vi "Realtime Curve Fitting.vi"() -> ()   [LabVIEW 2020]
panel:
  in  "Simulated Peak Width":dbl=1.5
  out "Fitted Peaks Widths":dbl(graph)=3.01437
  in  "stop":bool
  in  "Milliseconds to wait for Origin to Fit":u32=1000
  # "This example shows how to connect to Origin to do fitting on the simulated Gaussian peaks. And then show the dyamic changed widths of the peaks on the chart.\nThe simulated Gaussian peak is sent over to an Origin Analysis Template and the width of the peak is then brough back.\n\nBefore run this Vi, you can set the width of the simulated peak and the time to wait for Origin to Fit."
  # "Note: Random variation is also added."
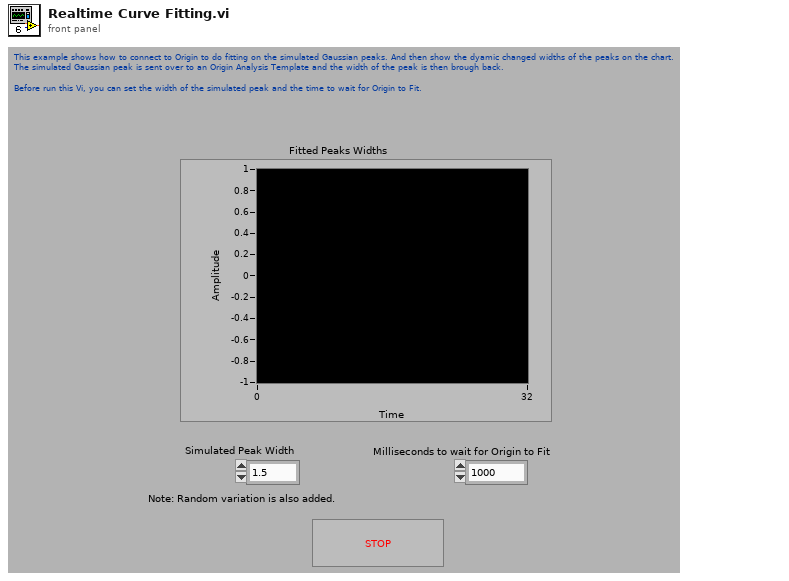
[diagram p1: front panel]
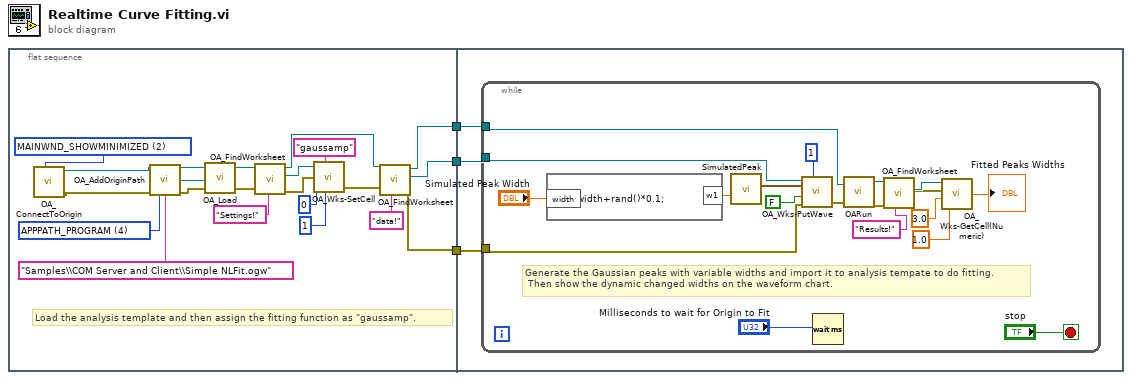
[diagram p0: block diagram]
diagram:
  n1 = flat-sequence {
    tunnel: [w16] -> w3
    tunnel: [w4] -> w2
    tunnel: [w15] -> w1
    tunnel: w3 -> [w28]
    tunnel: w2 -> [w27]
    tunnel: w1 -> [w26]
    frame #0 {
      w17 = 2 items=["MAINWND_HIDE"=0, "MAINWND_SHOW"=1, "MAINWND_SHOWMINIMIZED"=2, "MAINWND_SHOWMAXIMIZED"=3, "MAINWND_SHOW_BRING_TO_FRONT"=100] ("Visible")
      w23 = 4 items=["APPPATH_USER"=2, "APPPATH_GROUP"=3, "APPPATH_PROGRAM"=4] ("Type")
      # "Load the analysis template and then assign the fitting function as \"gaussamp\"."
      n2 = call "OA_ConnectToOrigin.vi"("Visible"=w17) -> ("error out"=w24:errorcluster, "Origin.IOApplication"=w25:refnum<k7>)  [unwired: 7 in]
      n3 = call "OA_AddOriginPath.vi"("Origin.IOApplication"=w25, "error in (no error)"=w24, "Type"=w23, "Filename"="Samples\\COM Server and Client\\Simple NLFit.ogw") -> ("Origin.IOApplication"=w21:refnum<k7>, "path out"=w20:path, "error out"=w19:errorcluster)  [unwired: 9 in]
      n4 = call "OA_Load.vi"("error in (no error)"=w19, "Path"=w20, "Origin.IOApplication"=w21) -> ("error out"=w13:errorcluster, "Origin.IOApplication"=w14:refnum<k7>)  [unwired: 1 out]
      n5 = call "OA_FindWorksheet.vi"("Name"="Settings!", "error in (no error)"=w13, "Origin.IOApplication"=w14) -> ("error out"=w7:errorcluster, "Origin.Worksheet"=w8:refnum<k7>, "Origin.IOApplication"=w6:refnum<k7>)  [unwired: 6 in]
      n6 = call "OA_Wks-SetCell.vi"("Origin.Worksheet"=w8, "Data"="gaussamp", "error in (no error)"=w7, "r1"=0, "c1"=1) -> ("error out"=w5:errorcluster)  [unwired: 2 out]
      n7 = call "OA_FindWorksheet.vi"("Name"="data!", "error in (no error)"=w5, "Origin.IOApplication"=w6) -> ("error out"=w4:errorcluster, "Origin.Worksheet"=w16:refnum<k7>, "Origin.IOApplication"=w15:refnum<k7>)  [unwired: 6 in]
    }
    frame #1 {
      n8 = while {
        tunnel: w28 -> [w47]
        tunnel: w27 -> [w46]
        tunnel: w26 -> [w40]
        stop <- "stop" stop-if-true
        # "Generate the Gaussian peaks with variable widths and import it to analysis tempate to do fitting.\n Then show the dynamic changed widths on the waveform chart."
        n9 = formula code="w1=width+rand()*0.1;"("width"="Simulated Peak Width") -> ("w1"=w39:dbl)
        n10 = call "SimulatedPeak.vi"("Width"=w39) -> ("Simulated Peak"=w44:waveform(dbl))  [unwired: 9 in]
        n11 = call "OA_Wks-PutWave.vi"("Origin.Worksheet"=w47, "Dynamic Data"=w44, "Append to existing data in column"=FALSE, "error in (no error)"=w46, "First Col Index"=1) -> ("error IO"=w30:errorcluster)  [unwired: 1 in, 1 out]
        n12 = Wait (ms)(milliseconds to wait="Milliseconds to wait for Origin to Fit") -> ()  [unwired: 1 out]
        n13 = call "OARun.vi"("Origin.IOApplication"=w40, "Error IO"=w30) -> ("Origin.IOApplication"=w35:refnum<k7>, "Error IO Out"=w36:errorcluster)  [unwired: 1 out]
        n14 = call "OA_FindWorksheet.vi"("Name"="Results!", "error in (no error)"=w36, "Origin.IOApplication"=w35) -> ("error out"=w33:errorcluster, "Origin.Worksheet"=w34:refnum<k7>)  [unwired: 6 in, 1 out]
        n15 = call "OA_Wks-GetCell(Numeric).vi"("c1"=1.0, "r1"=3.0, "error in (no error)"=w33, "Origin.Worksheet"=w34) -> ("Data"=→"Fitted Peaks Widths":dbl)  [unwired: 2 out]
      }
    }
  }
